vi "Append Text Table to Report.vi"(0 "report in":refnum<class "ooCalc.lvclass">, 1 "column width (1)":dbl=1.0 format="%.2f", 2 "measurement system":u16(ring)=2 caption="measurement system for column width (Default)" items=["US", "Metric", "Default"], 3 "MS Office parameters":T2, 5 "column headers":string[](array[string]), 7 "row headers":string[](array[string]), 9 "text data":string[][](array[string]), 11 "error in (no error)":errorcluster, 13 "separate page?":bool, 14 "show grid lines":bool=TRUE) -> (4 "report out":refnum<class "ooCalc.lvclass">, 8 "range (wd) - start (xl)":T1, 10 "end (xl)":cluster{"row (xl) ":i32, "col (xl) ":i32}, 15 "error out":errorcluster)   [LabVIEW 2009, in "ooCalc.lvclass"]
doc: "Appends a 2D array to a report as a table with the given column width. You can use this polymorphic VI to append an array of strings or numbers. The data type you wire to the <B>text data</B> input determines the polymorphic instance to use."
uses:
  ooCalc.lvclass
  ooCalc.lvclass/ooCalc.ctl
  C:/Projets/LAVAG/OpenOfficeRGT/AODL/DLLs/AODL.dll
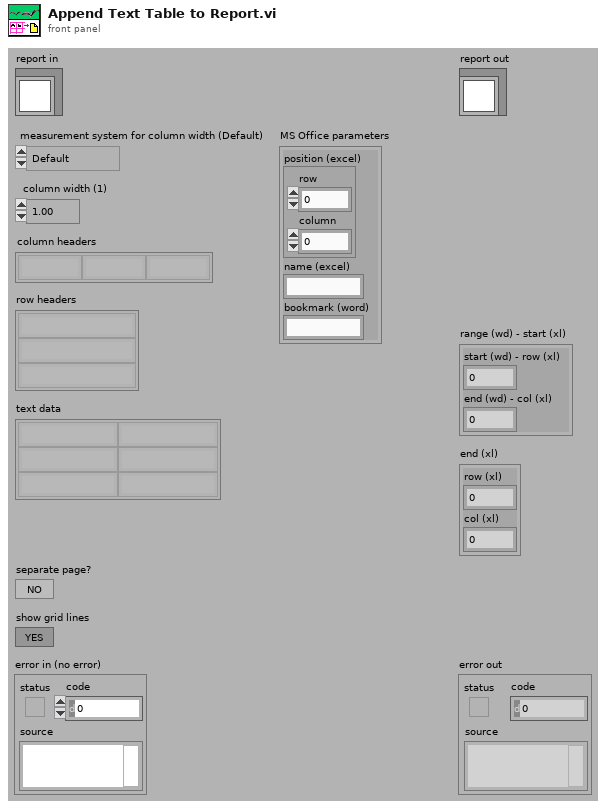
[diagram p1: front panel]
types:
  T1 = cluster{"start (wd) - row (xl) ":i32, "end (wd) - col (xl) ":i32}
  T2 = cluster{"position (excel)":cluster{"row":i32, "column":i32}, "name (excel)":string, "bookmark (word)":string}
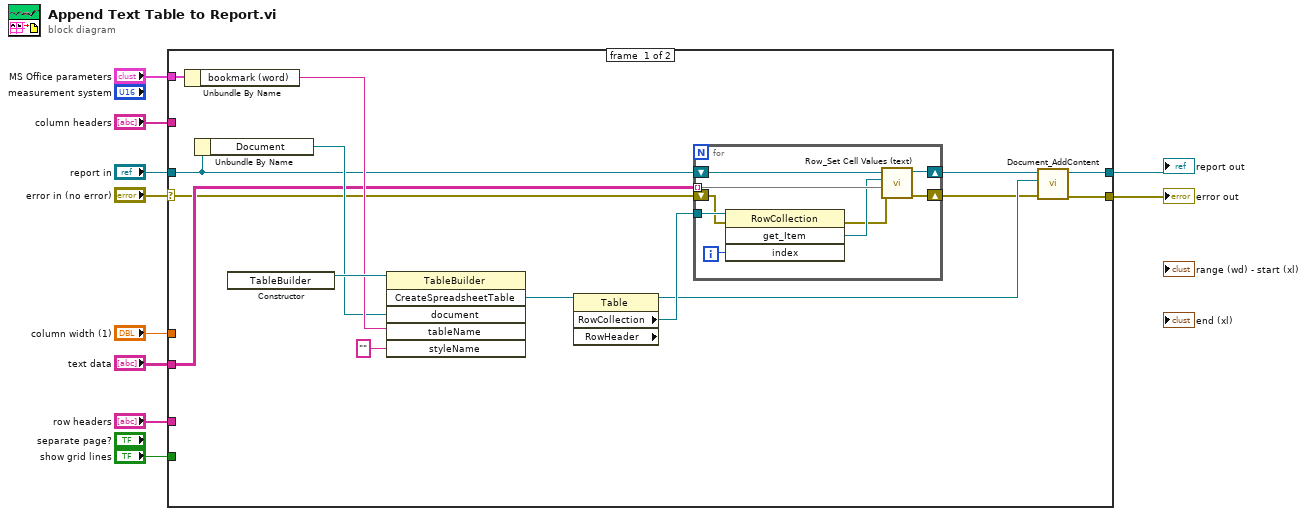
[diagram p0: block diagram]
diagram:
  n1 = case shown="No Error" "error in (no error)" {
    selector: "error in (no error)" -> [w11 w35]
    tunnel: [w18 w35] -> w9
    tunnel: "report in" -> [w17 w36]
    tunnel: [w19 w36] -> w7
    tunnel: "show grid lines" -> [_ _]
    tunnel: "text data" -> [w15 _]
    tunnel: "column width (1)" -> [_ _]
    tunnel: "MS Office parameters" -> [w24 _]
    tunnel: "column headers" -> [_ _]
    tunnel: "row headers" -> [_ _]
    frame #0 {
      n2 = Unbundle By Name(w24) -> ("bookmark (word)"=w23:string)
      n3 = Unbundle By Name(w17) -> ("Document"=w21:refnum<k24>)
      n4 = constructor class="TableBuilder"() -> (reference out=w25:refnum<k24>)  [unwired: 3 in, 2 out]
      n5 = invoke class="TableBuilder" method="CreateSpreadsheetTable"(reference=w25, "document"=w21, "tableName"=w23, "styleName"="") -> ("CreateSpreadsheetTable"=w20:refnum<k24>)  [unwired: 2 in, 5 out]
      n6 = property class="Table" props=["RowCollection", "RowHeader"](reference=w20) -> (reference out=w13:refnum<k24>, "RowCollection"=w14:refnum<k24>)  [unwired: 1 in, 2 out]
      n7 = for {
        shift-right: [w33] -> w16
        shift-left: w17 -> [w34]
        tunnel: w15 -> [w32] mode=indexing
        tunnel: w14 -> [w30]
        shift-right: [w27] -> w12
        shift-left: w11 -> [w26]
        i -> [w31]
        n8 = invoke class="RowCollection" method="get_Item"(reference=w30, error in=w26, "index"=w31) -> (error out=w28:errorcluster, "get_Item"=w29:refnum<k24>)  [unwired: 1 in, 2 out]
        n9 = call-dynamic "Row_Set Cell Values (text).vi"("error in (no error)"=w28, "text data (row)"=w32, "Row"=w29, "ooWriter in"=w34) -> ("error out"=w27:errorcluster, "ooWriter out"=w33:refnum<class "ooCalc.lvclass">)  [unwired: 6 in]
      }
      n10 = call-dynamic "Document_AddContent.vi"("error in (no error)"=w12, "Content"=w13, "ooWriter in"=w16) -> ("error out"=w18:errorcluster, "ooWriter out"=w19:refnum<class "ooCalc.lvclass">)  [unwired: 7 in]
    }
    frame #1 {
    }
  }
  "error out" <- w9
  "report out" <- w7
